vi "Test 1.vi"() -> ()   [LabVIEW 2020, in "Scratchpad.lvlib"]
uses:
  Scratchpad.lvlib
  Test Caller/Test Caller/Test Caller.lvclass
  Artifex/Actor/Actor.lvclass
panel:
  out "error out":errorcluster
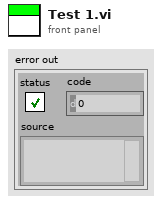
[diagram p1: front panel]
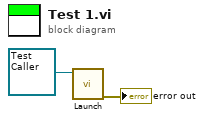
[diagram p0: block diagram]
diagram:
  n1 = call "Launch.vi"("Actor in"=refnum<class "Test Caller.lvclass"> refnum ("Scratchpad.lvlib:Test Caller.lvlib:Test Caller.lvclass")) -> ("error out"=→"error out":errorcluster)  [unwired: 9 in, 1 out]
